vi "DSF.Engine.Transceiver.Initialize.vi"(8 "error in (no error)":errorcluster, 9 "transceiver settings":T1, 10 "Transfer Groups Configurations":refnum<class "DSF.Shared.Configuration.Transfer Group.lvclass">[](array[class]), 11 "UDP Transceiver in":refnum<class "DSF.Transceiver.UDP.lvclass">) -> (0 "error out":errorcluster, 3 "UDP Transceiver out":refnum<class "DSF.Transceiver.UDP.lvclass">)   [LabVIEW 2017, in "DSF.Transceiver.UDP.lvlib" / "DSF.Transceiver.UDP.lvclass"]
uses:
  DSF.Transceiver.UDP.lvclass
  DSF Core/Built/Engine/DSF.Engine.lvlibp/Shared/Classes/Transfer Group/DSF.Shared.Configuration.Transfer Group.lvclass
  DSF Core/Built/Engine/DSF.Engine.lvlibp/DSF Configuration API/1.0.0/Public/Controls/DSF Settings Info.ctl
  DSF.Transceiver.UDP.lvclass/DSF.Transceiver.UDP.ctl
  DSF Core/Built/Engine/DSF.Engine.lvlibp/DSF Configuration API/1.0.0/DSF Configuration API.lvlib
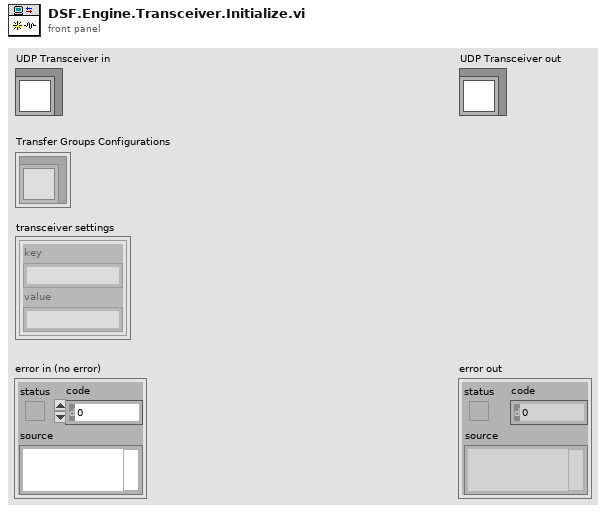
[diagram p1: front panel]
types:
  T1 = typedef "DSF.Engine.lvlibp/DSF Configuration API.lvlib/DSF Settings Info.ctl" = cluster{"key":string, "value":string}[]
  T2 = typedef "DSF.Transceiver.UDP.lvlib/DSF.Transceiver.UDP.lvclass/DSF.Transceiver.UDP.Parameters.Transfer Group.ctl" = cluster{"Rx":T3, "Tx":T5}
  T3 = typedef "DSF.Transceiver.UDP.lvlib/DSF.Transceiver.UDP.lvclass/DSF.Transceiver.UDP.Parameters.Transfer Group.Rx.ctl" = cluster{"Transfers Rx":T4[], "max size":i32}
  T4 = typedef "DSF.Transceiver.UDP.lvlib/DSF.Transceiver.UDP.lvclass/DSF.Transceiver.UDP.Parameters.Transfer.Rx.ctl" = cluster{"timeout":i32, "source address":u32, "source port":u16}
  T5 = typedef "DSF.Transceiver.UDP.lvlib/DSF.Transceiver.UDP.lvclass/DSF.Transceiver.UDP.Parameters.Transfer Group.Tx.ctl" = cluster{"Transfers Tx":T6[]}
  T6 = typedef "DSF.Transceiver.UDP.lvlib/DSF.Transceiver.UDP.lvclass/DSF.Transceiver.UDP.Parameters.Transfer.Tx.ctl" = cluster{"destination port":u16, "destination address":u32}
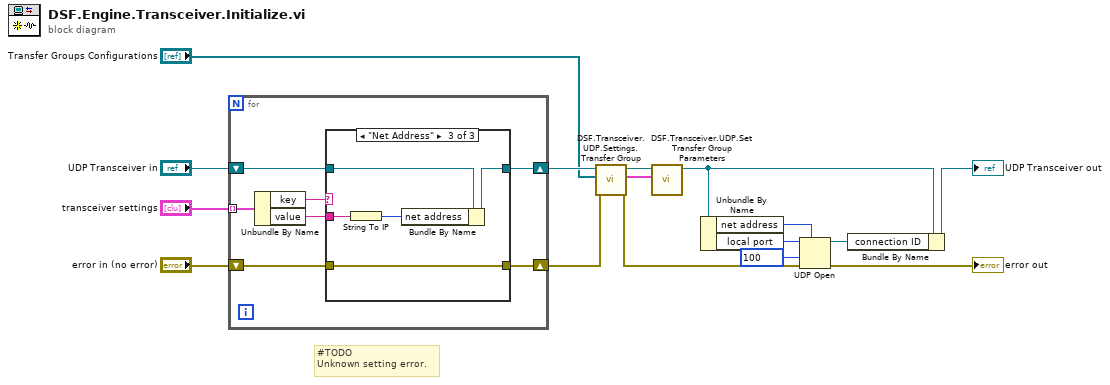
[diagram p0: block diagram]
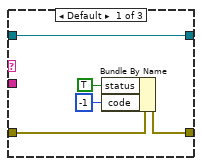
[diagram p2: hidden frame]
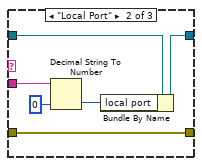
[diagram p3: hidden frame]
diagram:
  # "#TODO\nUnknown setting error."
  n1 = for {
    tunnel: "transceiver settings" -> [w23] mode=indexing
    shift-right: [w19] -> w12
    shift-left: "UDP Transceiver in" -> [w20]
    shift-right: [w17] -> w10
    shift-left: "error in (no error)" -> [w18]
    n2 = Unbundle By Name(w23) -> ("key"=w22:string, "value"=w21:string)
    n3 = case shown="\"Net Address\"" w22 {
      tunnel: w21 -> [_ w33 w36]
      tunnel: w20 -> [w28 w32 w39]
      tunnel: [w28 w31 w38] -> w19
      tunnel: w18 -> [w27 w30 w37]
      tunnel: [w26 w30 w37] -> w17
      frame Default {
        n4 = Bundle By Name(cluster=w27, "status"=TRUE, "code"=-1) -> (w26:errorcluster)
      }
      frame "Local Port" {
        n5 = Decimal String To Number(string=w33, default (0L)=u16 0 ("default (0 I32)")) -> (number=w29:u16)  [unwired: 1 in, 1 out]
        n6 = Bundle By Name(cluster=w32, "local port"=w29) -> (w31:refnum<class "DSF.Transceiver.UDP.lvclass">)
      }
      frame "Net Address" {
        n7 = String To IP(1:w36) -> (0:w35:u32)
        n8 = Bundle By Name(cluster=w39, "net address"=w35) -> (w38:refnum<class "DSF.Transceiver.UDP.lvclass">)
      }
    }
  }
  n9 = call "DSF.Transceiver.UDP.Settings.Transfer Group.vi"("error in (no error)"=w10, "Transfer Groups Configurations"="Transfer Groups Configurations", "UDP Transceiver in"=w12) -> ("error out"=w8:errorcluster, "Transfer Group parameters"=w15:T2[], "UDP Transceiver out"=w16:refnum<class "DSF.Transceiver.UDP.lvclass">)  [unwired: 6 in]
  n10 = call "DSF.Transceiver.UDP.Set Transfer Group Parameters.vi"("Transfer Group parameters"=w15, "UDP Transceiver in"=w16) -> ("UDP Transceiver out"=w7:refnum<class "DSF.Transceiver.UDP.lvclass">)  [unwired: 9 in]
  n11 = Unbundle By Name(w7) -> ("net address"=w1:u32, "local port"=w6:u16)
  n12 = UDP Open(7:w1, 8:w8, 9:100 ("timeout ms (25000)"), 11:w6) -> (port=w4:refnum<k16>, 0:→"error out":errorcluster)  [unwired: 1 in, 1 out]
  n13 = Bundle By Name(cluster=w7, "connection ID"=w4) -> (→"UDP Transceiver out":refnum<class "DSF.Transceiver.UDP.lvclass">)
